vi "Panel Origin Zero.vi"(8 "error in":errorcluster, 11 "Last Level":i32=1) -> (0 "error out":errorcluster)   [LabVIEW 2020]
uses:
  <vilib>/Utility/miscctls.llb/LVPointTypeDef.ctl
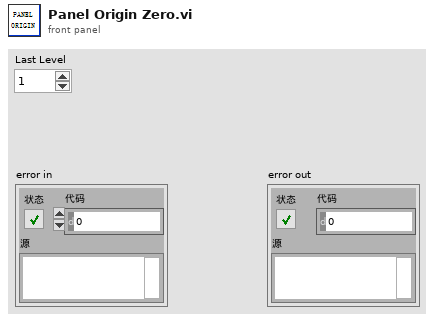
[diagram p1: front panel]
types:
  T1 = typedef "LVPointTypeDef.ctl" = cluster{"Horizontal":i16, "Vertical":i16}
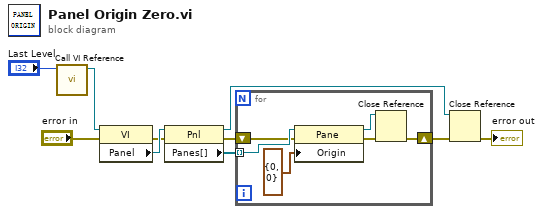
[diagram p0: block diagram]
diagram:
  n1 = call "Call VI Reference.vi"("last level"="Last Level") -> ("vi reference out"=w9:refnum<vi>)  [unwired: 9 in, 1 out]
  n2 = property class="VI"(reference=w9, error in="error in") -> (error out=w5:errorcluster, "Panel"=w8:refnum<vi>)  [unwired: 1 out]
  n3 = property class="Pnl"(reference=w8, error in=w5) -> (reference out=w3:refnum<vi>, error out=w4:errorcluster, "Panes[]"=w7:refnum<vi>[])
  n4 = for {
    tunnel: w7 -> [w16] mode=indexing
    shift-right: [w12] -> w2
    shift-left: w4 -> [w15]
    n5 = property class="Pane"(reference=w16, error in=w15, "Origin"=T1 {"Horizontal"=0, "Vertical"=0} ("原点")) -> (reference out=w13:refnum<vi>, error out=w14:errorcluster)
    n6 = Close Reference(reference=w13, error in (no error)=w14) -> (error out=w12:errorcluster)
  }
  n7 = Close Reference(reference=w3, error in (no error)=w2) -> (error out=→"error out":errorcluster)
